vi "File Page - Edit Waveform Table.vi"(4 "New String":string, 6 "Coords":T2, 8 "error in (no error)":errorcluster, 9 "Item Ref in":T1 format="%.0x", 10 "Events in":string[](array[string]), 11 "File Waveforms in":T3 {"Node Refs" format="%.0x"}) -> (0 "error out":errorcluster, 1 "Discard?":bool, 2 "Events out":string[](array[string]), 3 "File Waveforms out":T3 {"Node Refs" format="%.0x"})   [LabVIEW 2015, in "Waveform Data Logger System Explorer.lvlib"]
uses:
  Waveform Data Logger System Explorer.lvlib
  Types/File - Waveforms.ctl
  <vilib>/NI Veristand/Custom Device API/Custom Device Item Ref.ctl
  <vilib>/Utility/miscctls.llb/LVRowAndColumnTypeDef.ctl
  Shared/Globals/Property Strings.vi
  <vilib>/NI Veristand/Custom Device API/Set Item Property (String Array).vi
  <vilib>/NI Veristand/Custom Device API/Set Item Property (U32 Array).vi
  <vilib>/NI VeriStand/Custom Device API/Custom Device API.lvlib
  Shared/Waveform Data Logger Shared.lvlib
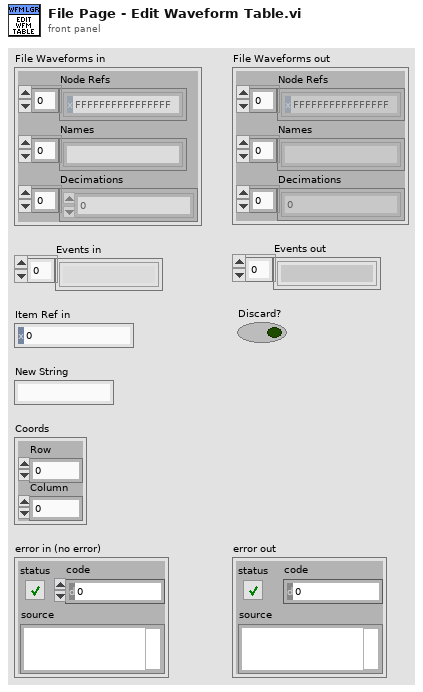
[diagram p1: front panel]
types:
  T1 = typedef "Custom Device API.lvlib/Custom Device Item Ref.ctl" = u64
  T2 = typedef "LVRowAndColumnTypeDef.ctl" = cluster{"Row":i32, "Column":i32}
  T3 = typedef "Waveform Data Logger System Explorer.lvlib/File - Waveforms.ctl" = cluster{"Node Refs":T1[], "Names":string[], "Decimations":u32[]}
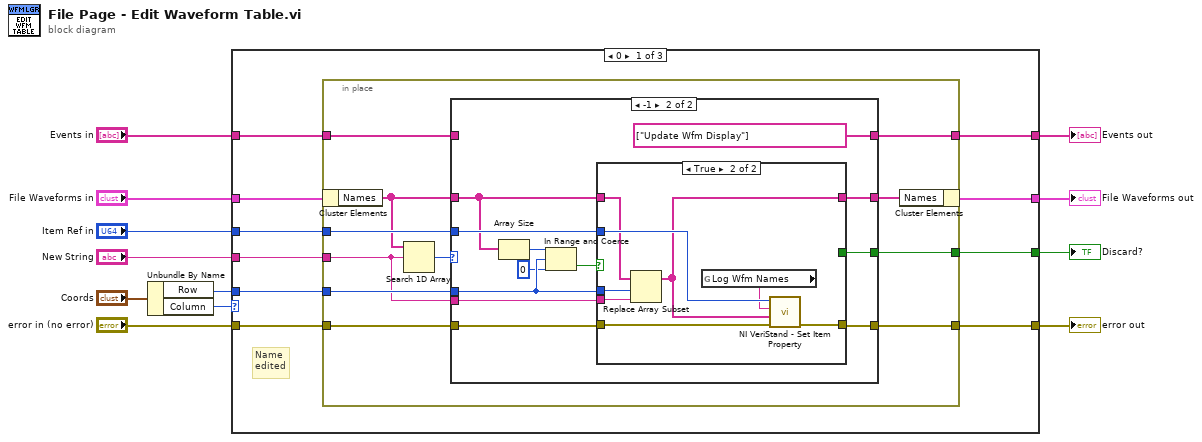
[diagram p0: block diagram]
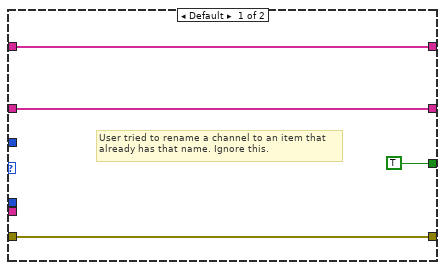
[diagram p2: hidden frame]
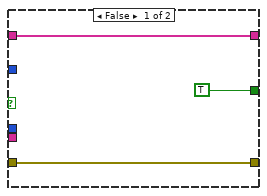
[diagram p3: hidden frame]
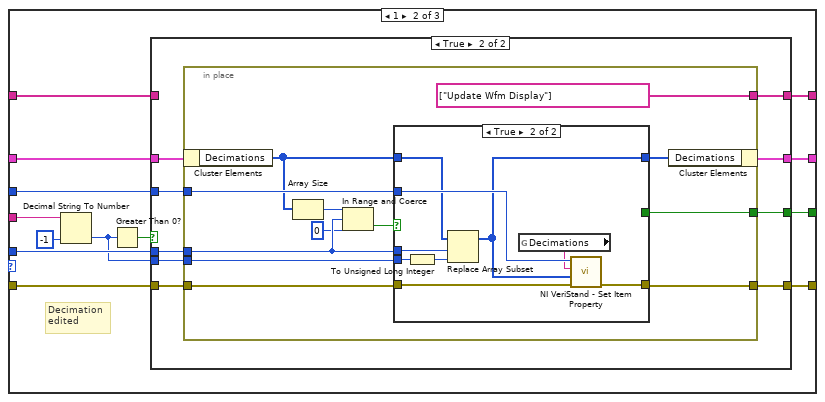
[diagram p4: hidden frame]
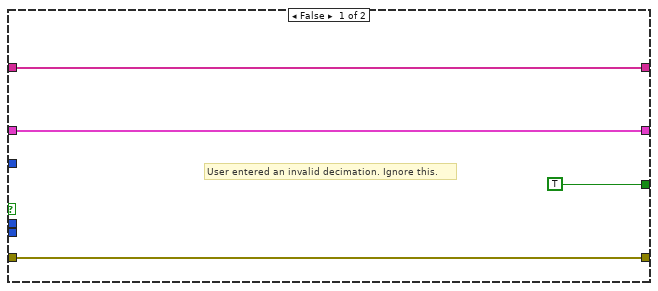
[diagram p5: hidden frame]
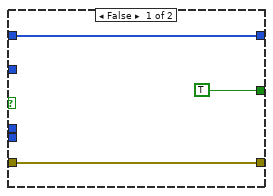
[diagram p6: hidden frame]
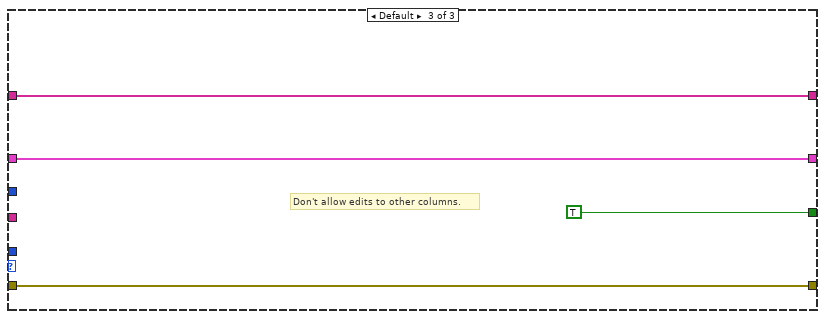
[diagram p7: hidden frame]
diagram:
  n1 = Unbundle By Name("Coords") -> ("Row"=w2:i32, "Column"=w3:i32)
  n2 = case shown="0" w3 {
    tunnel: w2 -> [w19 w70 _]
    tunnel: [w22 w73 TRUE] -> w12
    tunnel: "New String" -> [w18 w65 _]
    tunnel: "Events in" -> [w20 w71 w113]
    tunnel: [w21 w72 w113] -> w6
    tunnel: "error in (no error)" -> [w17 w69 w112]
    tunnel: "Item Ref in" -> [w16 w68 _]
    tunnel: [w15 w67 w112] -> w11
    tunnel: "File Waveforms in" -> [w14 w62 w111]
    tunnel: [w13 w61 w111] -> w1
    frame 0 {
      # "Name\nedited"
      n3 = in-place {
        in-place-border: [w32] -> w22
        in-place-border: [w31] -> w21
        in-place-border: w20 -> [w30]
        in-place-border: w19 -> [w29]
        in-place-border: w18 -> [w28]
        in-place-border: w17 -> [w27]
        in-place-border: w16 -> [w26]
        in-place-border: [w25] -> w15
        n4 = in-place-cluster #1(w14) -> ("Names"=w24:string[])
        n5 = Search 1D Array(1D array=w24, element=w28) -> (index of element=w33:i32)  [unwired: 1 in]
        n6 = case shown="-1" w33 {
          tunnel: [TRUE w38] -> w32
          tunnel: [w36 string[] ["Update Wfm Display"]] -> w31
          tunnel: w30 -> [w36 _]
          tunnel: [w35 w45] -> w23
          tunnel: w24 -> [w35 w43]
          tunnel: w29 -> [_ w41]
          tunnel: w28 -> [_ w48]
          tunnel: w27 -> [w34 w47]
          tunnel: w26 -> [_ w46]
          tunnel: [w34 w44] -> w25
          frame Default {
            # "User tried to rename a channel to an item that\nalready has that name. Ignore this."
          }
          frame -1 {
            n7 = Array Size(array=w43) -> (size(s)=w42:i32)
            n8 = In Range and Coerce(upper limit=w42, x=w41, lower limit=0) -> (In Range?=w40:bool)  [unwired: 1 out]
            n9 = case shown="True" w40 {
              tunnel: w41 -> [_ w60]
              tunnel: w48 -> [_ w59]
              tunnel: w47 -> [w51 w58]
              tunnel: w46 -> [_ w57]
              tunnel: [w52 w56] -> w45
              tunnel: [w51 w55] -> w44
              tunnel: w43 -> [w52 w54]
              tunnel: [TRUE _] -> w38
              frame False {
              }
              frame True {
                n10 = Replace Array Subset(array=w54, new element=w59, index=w60) -> (w56:string[])
                n11 = global read "Property Strings.vi" "Log Wfm Names"() -> (w53:string)
                n12 = call-poly <vilib>:"NI VeriStand - Set Item Property.vi"("error in (no error)"=w58, "Value"=w56, "Property Name"=w53, "Item Ref in"=w57) -> ("error out"=w55:errorcluster)  [unwired: 7 out]
              }
            }
          }
        }
        n13 = in-place-cluster #1("Names"=w23) -> (w13:T3)
      }
    }
    frame 1 {
      # "Decimation\nedited"
      n14 = Decimal String To Number(string=w65, default (0L)=-1 ("default (0 I32)")) -> (number=w63:i32)  [unwired: 1 in, 1 out]
      n15 = Greater Than 0?(x=w63) -> (x > 0?=w64:bool)
      n16 = case shown="True" w64 {
        tunnel: [TRUE w82] -> w73
        tunnel: [w76 w78] -> w72
        tunnel: w71 -> [w76 _]
        tunnel: w70 -> [_ w83]
        tunnel: w69 -> [w75 w86]
        tunnel: w68 -> [_ w85]
        tunnel: [w75 w84] -> w67
        tunnel: w63 -> [_ w81]
        tunnel: w62 -> [w74 w80]
        tunnel: [w74 w79] -> w61
        frame False {
          # "User entered an invalid decimation. Ignore this."
        }
        frame True {
          n17 = in-place {
            in-place-border: w86 -> [w98]
            in-place-border: w85 -> [w97]
            in-place-border: [w96] -> w84
            in-place-border: w83 -> [w94]
            in-place-border: [w91] -> w82
            in-place-border: w81 -> [w90]
            in-place-border: [string[] ["Update Wfm Display"]] -> w78
            n18 = in-place-cluster #2(w80) -> ("Decimations"=w89:u32[])
            n19 = Array Size(array=w89) -> (size(s)=w95:i32)
            n20 = In Range and Coerce(upper limit=w95, x=w94, lower limit=0) -> (In Range?=w93:bool)  [unwired: 1 out]
            n21 = case shown="True" w93 {
              tunnel: w94 -> [_ w110]
              tunnel: w98 -> [w101 w109]
              tunnel: w97 -> [_ w108]
              tunnel: [w101 w107] -> w96
              tunnel: [TRUE _] -> w91
              tunnel: w89 -> [w99 w105]
              tunnel: [w99 w104] -> w88
              tunnel: w90 -> [_ w103]
              frame False {
              }
              frame True {
                n22 = To Unsigned Long Integer(number=w103) -> (unsigned 32bit integer=w102:u32)
                n23 = Replace Array Subset(array=w105, new element=w102, index=w110) -> (w104:u32[])
                n24 = global read "Property Strings.vi" "Decimations"() -> (w106:string)
                n25 = call-poly <vilib>:"NI VeriStand - Set Item Property.vi"("error in (no error)"=w109, "Value"=w104, "Property Name"=w106, "Item Ref in"=w108) -> ("error out"=w107:errorcluster)  [unwired: 7 out]
              }
            }
            n26 = in-place-cluster #2("Decimations"=w88) -> (w79:T3)
          }
        }
      }
    }
    frame Default {
      # "Don't allow edits to other columns."
    }
  }
  "File Waveforms out" <- w1
  "Discard?" <- w12
  "error out" <- w11
  "Events out" <- w6
